vi "Main.vi"() -> ()   [LabVIEW 2018]
panel:
  in  "Air Dry Position Switch":bool
  in  "Main Wash Position Switch":bool
  in  "Under Body Wash Position Switch":bool
  in  "Economy Wash":bool
  in  "Deluxe Wash":bool
  out "Vehicle Out of Position":bool
  out "Air Dry":bool
  out "Clear Water Rinse":bool
  out "Main High Pressure Wash":bool
  out "Soap Aplication":bool
  out "Under Body Wash":bool
  in  "Stop":bool
  # "Purchase Selection"
  # "Car Wash Indicators"
  # "Car Wash Simulation Switches"
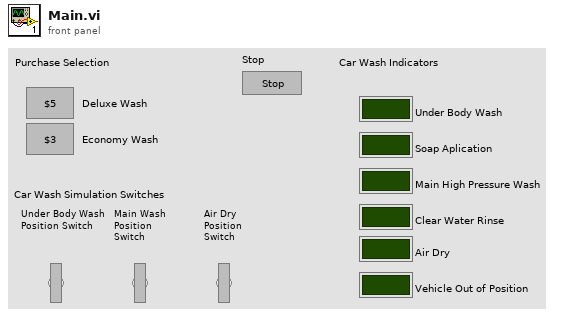
[diagram p1: front panel]
types:
  T1 = enum8{"Enabled", "Disabled", "Disabled and Grayed Out"}
  T2 = typedef "lista stnów.ctl" = enum16{"start", "ubderbody", "soap", "main", "main high", "clear water", "air", "air dry", "koniec"}
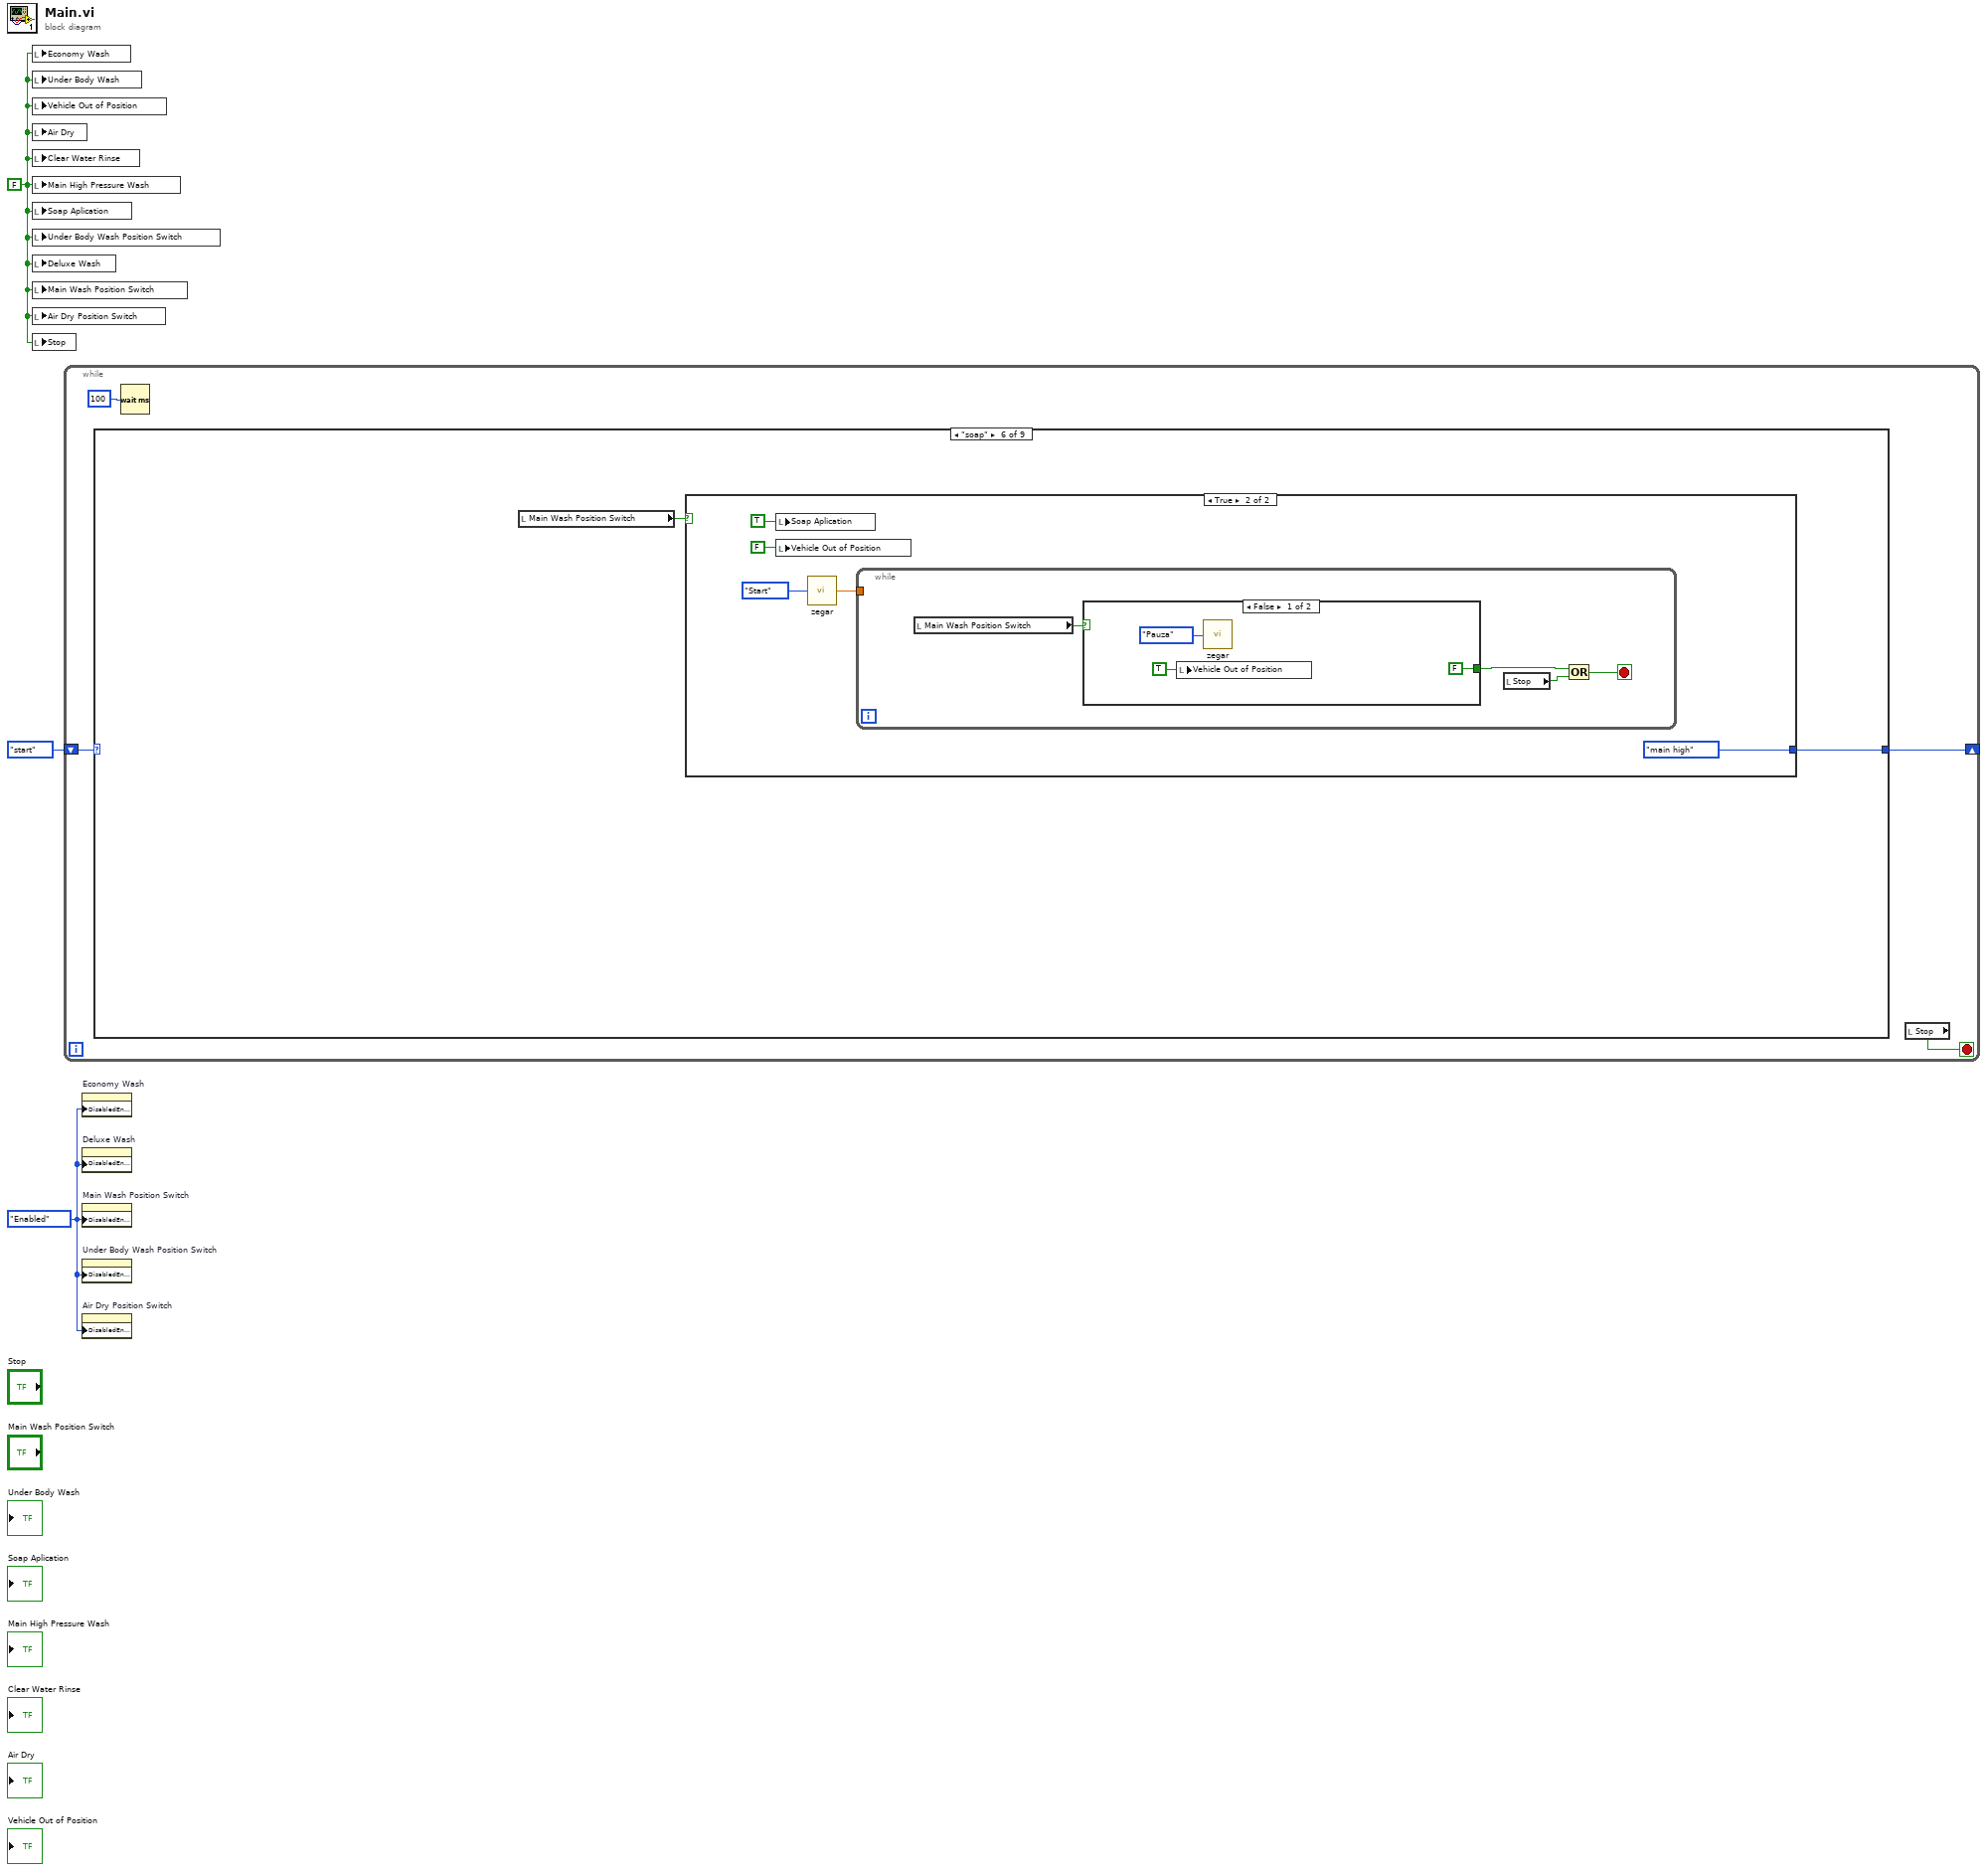
[diagram p0: block diagram]
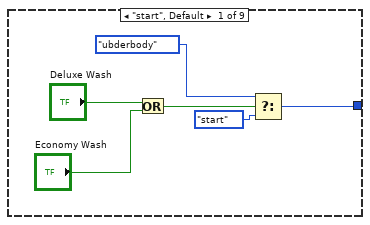
[diagram p2: hidden frame]
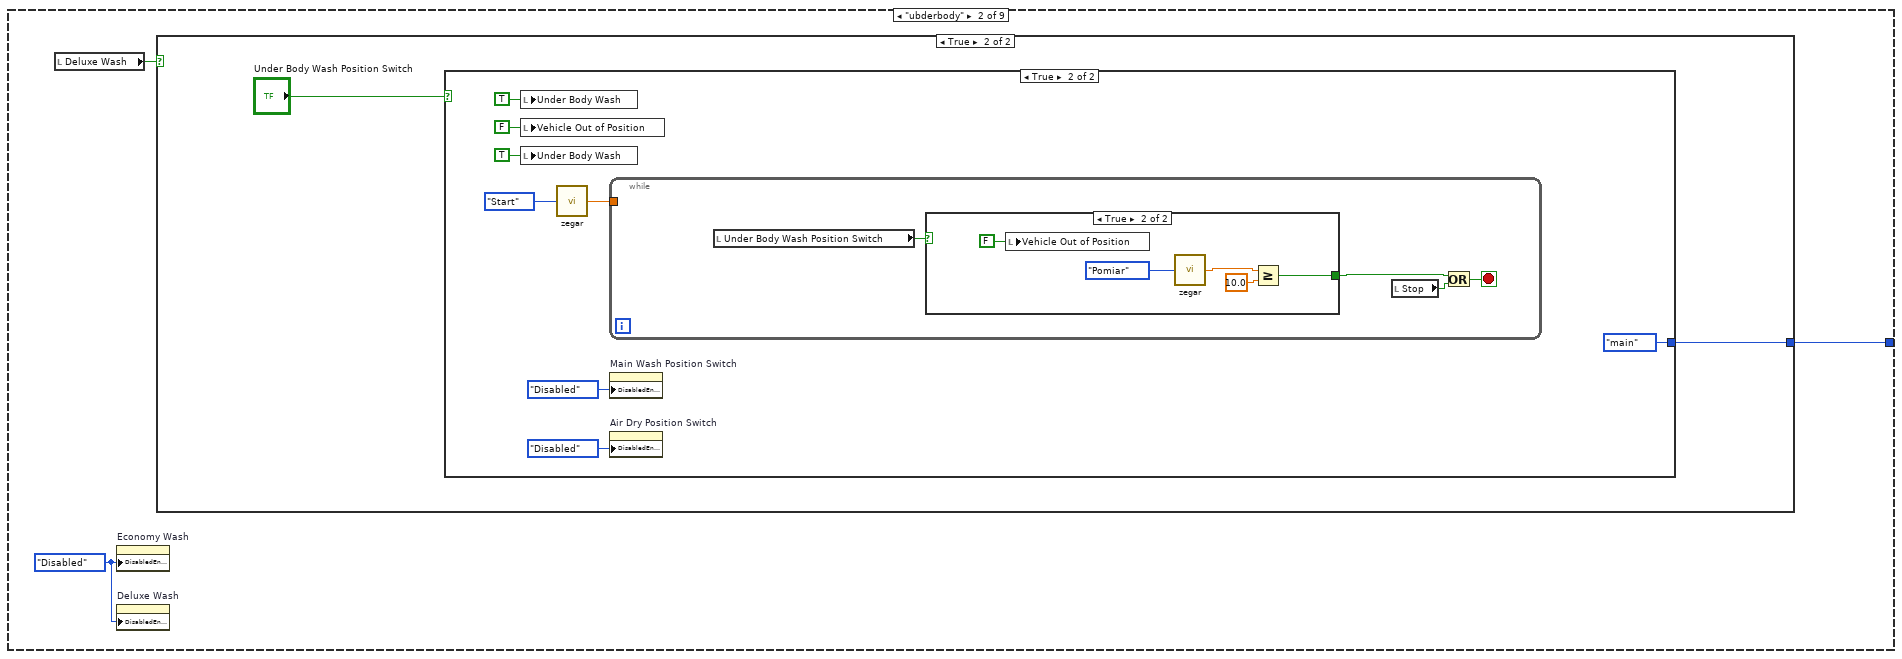
[diagram p3: hidden frame]
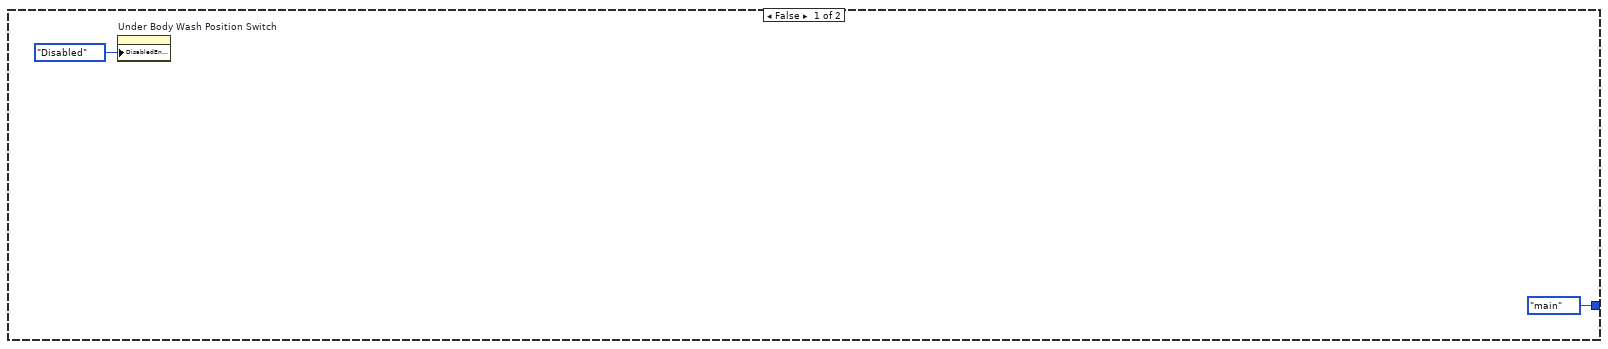
[diagram p4: hidden frame]
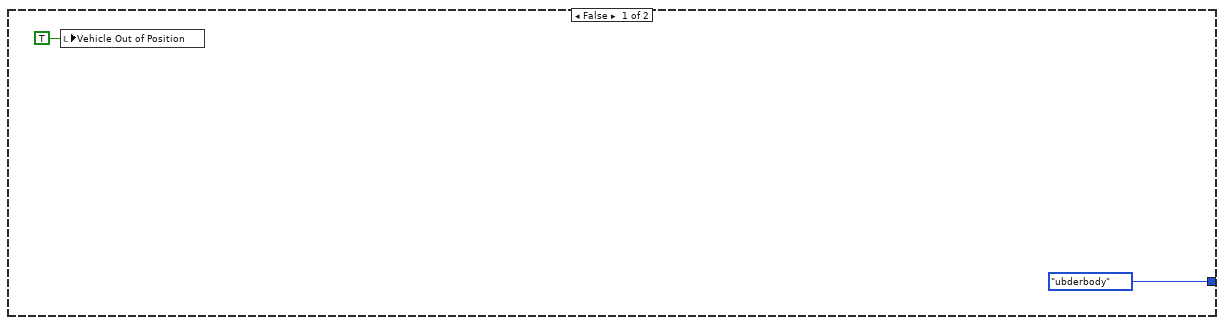
[diagram p5: hidden frame]
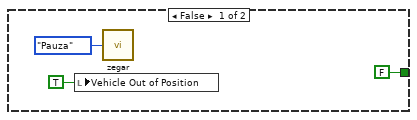
[diagram p6: hidden frame]
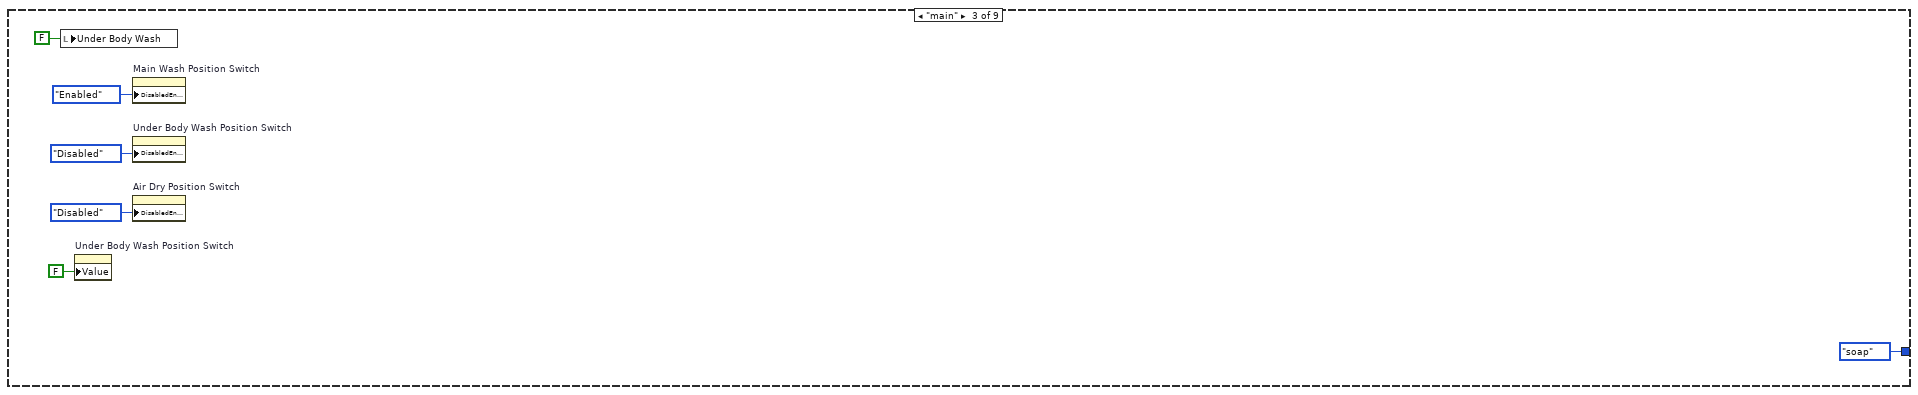
[diagram p7: hidden frame]
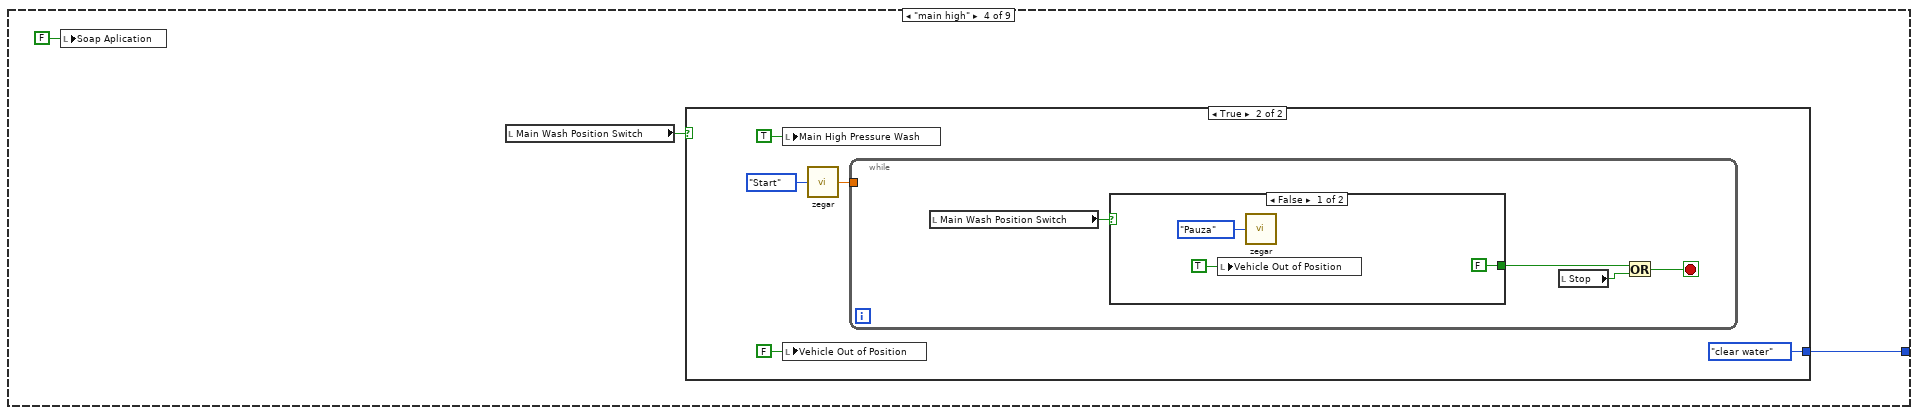
[diagram p8: hidden frame]
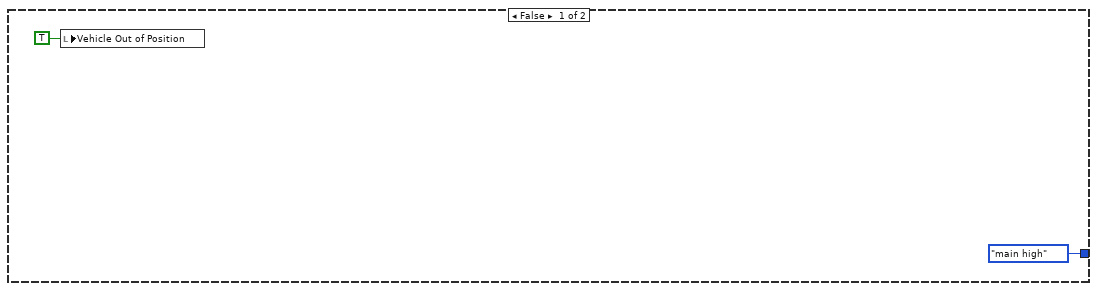
[diagram p9: hidden frame]
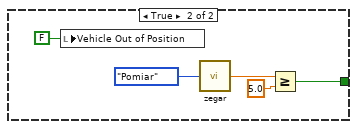
[diagram p10: hidden frame]
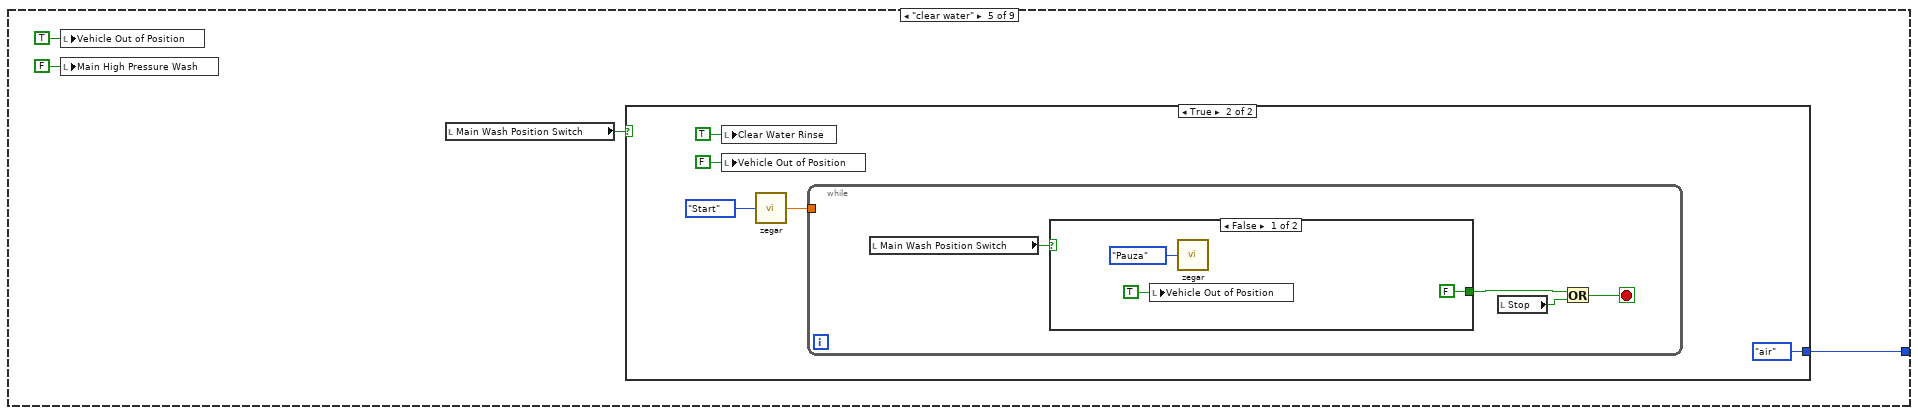
[diagram p11: hidden frame]
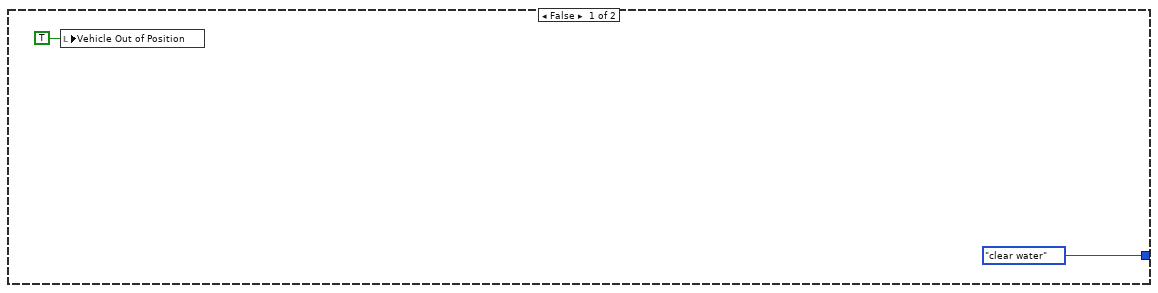
[diagram p12: hidden frame]
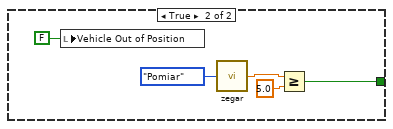
[diagram p13: hidden frame]
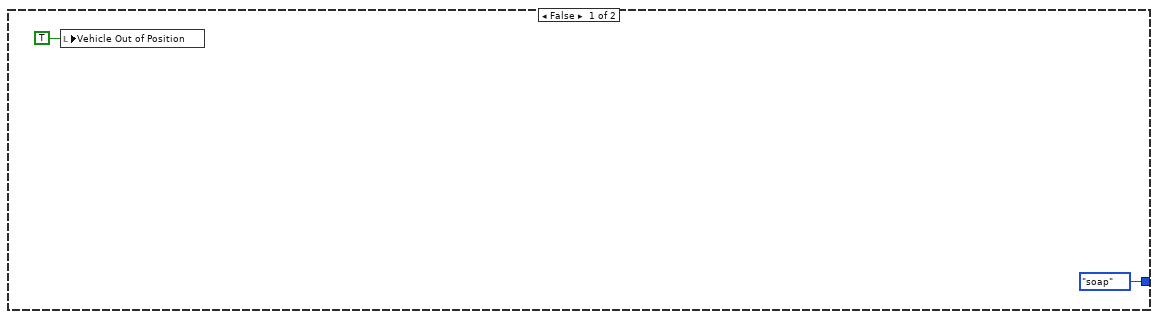
[diagram p14: hidden frame]
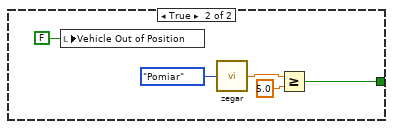
[diagram p15: hidden frame]
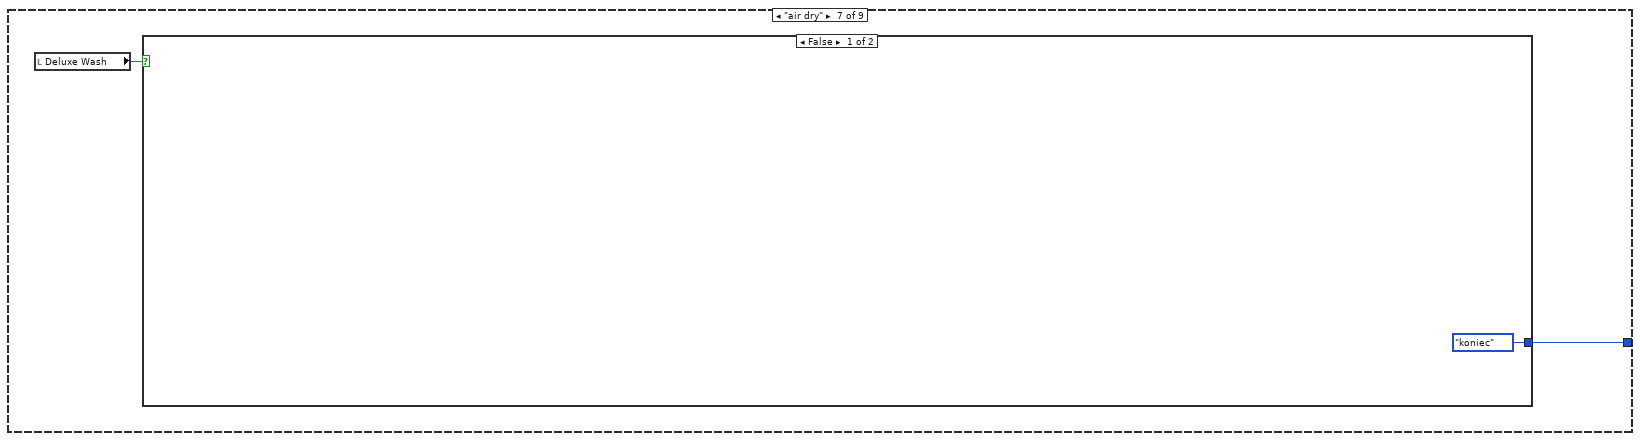
[diagram p16: hidden frame]
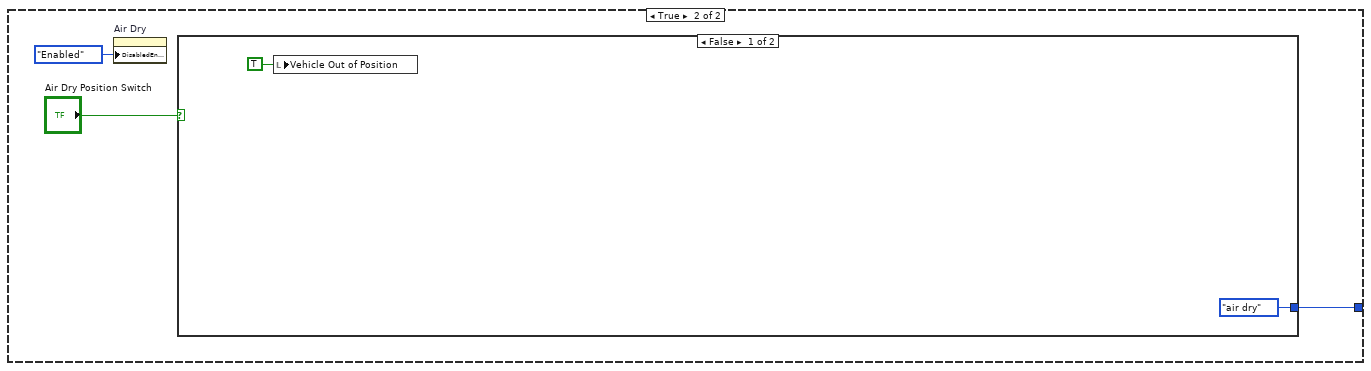
[diagram p17: hidden frame]
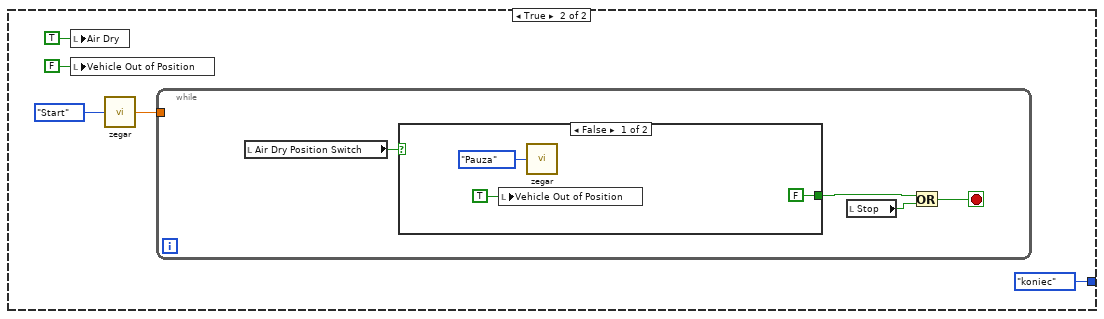
[diagram p18: hidden frame]
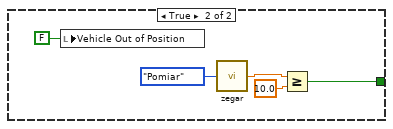
[diagram p19: hidden frame]
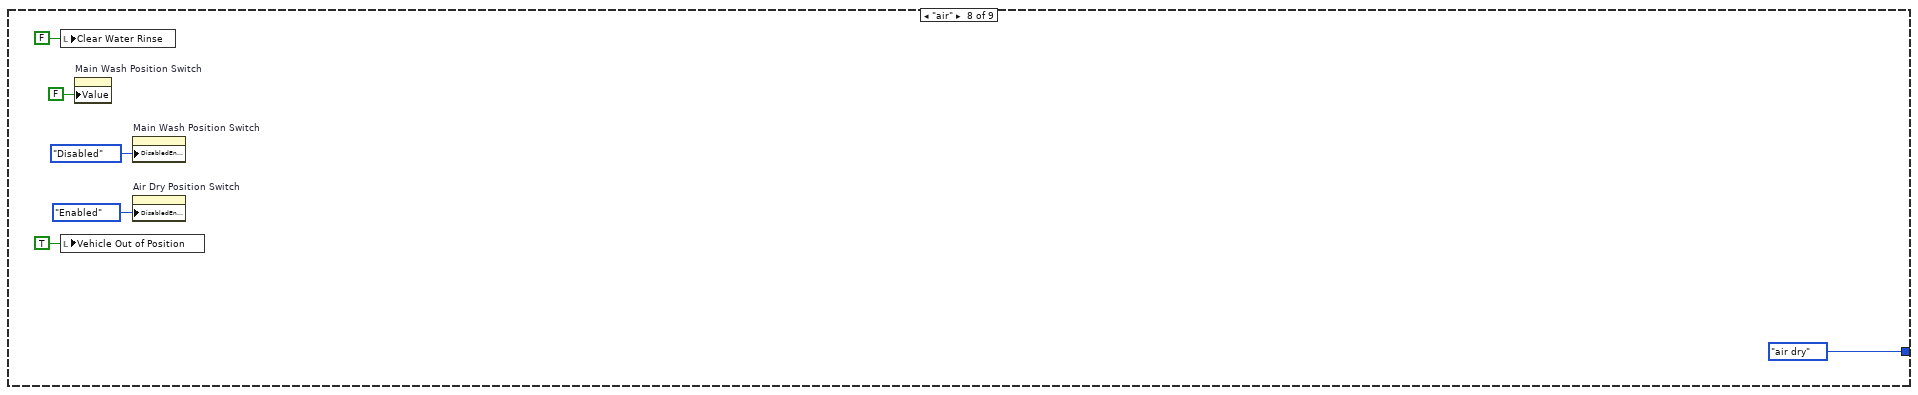
[diagram p20: hidden frame]
diagram:
  w1 = T1."Enabled" ("Disabled")
  w2 = FALSE
  n1 = local write "Economy Wash"(w2) -> ()
  n2 = local write "Under Body Wash"(w2) -> ()
  n3 = local write "Vehicle Out of Position"(w2) -> ()
  n4 = local write "Air Dry"(w2) -> ()
  n5 = local write "Clear Water Rinse"(w2) -> ()
  n6 = local write "Main High Pressure Wash"(w2) -> ()
  n7 = local write "Soap Aplication"(w2) -> ()
  n8 = local write "Under Body Wash Position Switch"(w2) -> ()
  n9 = local write "Deluxe Wash"(w2) -> ()
  n10 = local write "Main Wash Position Switch"(w2) -> ()
  n11 = local write "Air Dry Position Switch"(w2) -> ()
  n12 = local write "Stop"(w2) -> ()
  n13 = while {
    shift-right: [w5] -> _
    shift-left: lista_stnów."start" -> [w4]
    stop <- w7 stop-if-true
    n14 = case shown="\"soap\"" w4 {
      tunnel: [w8 w15 lista_stnów."soap" w49 w72 w94 w115 lista_stnów."air dry" lista_stnów."start"] -> w5
      frame "start", Default {
        n15 = Or(x="Deluxe Wash", y="Economy Wash") -> (x .or. y?=w11:bool)
        n16 = Select(t=lista_stnów."ubderbody", s=w11, f=lista_stnów."start") -> (s? t:f=w8:T2)
      }
      frame "ubderbody" {
        w14 = T1."Disabled" ("Disabled")
        n17 = local read "Deluxe Wash"() -> (w16:bool)
        n18 = property on="Economy Wash" class="Bool (strict)"("DisabledEnum"=w14) -> ()  [unwired: 2 in, 2 out]
        n19 = property on="Deluxe Wash" class="Bool (strict)"("DisabledEnum"=w14) -> ()  [unwired: 2 in, 2 out]
        n20 = case shown="True" w16 {
          tunnel: [lista_stnów."main" w19] -> w15
          frame False {
            n21 = property on="Under Body Wash Position Switch" class="Bool (strict)"("DisabledEnum"=T1."Disabled" ("Disabled")) -> ()  [unwired: 2 in, 2 out]
          }
          frame True {
            n22 = case shown="True" "Under Body Wash Position Switch" {
              tunnel: [lista_stnów."ubderbody" lista_stnów."main"] -> w19
              frame False {
                n23 = local write "Vehicle Out of Position"(TRUE ("Vehicle Out of Position 2")) -> ()
              }
              frame True {
                n24 = local write "Under Body Wash"(TRUE ("Under Body Wash")) -> ()
                n25 = local write "Vehicle Out of Position"(FALSE ("Vehicle Out of Position")) -> ()
                n26 = local write "Under Body Wash"(TRUE ("Under Body Wash")) -> ()
                n27 = call "zegar.vi"("zadanie"=enum16{"Start", "Pauza", "Pomiar"}."Start") -> ("x-y"=w26:dbl)
                n28 = while {
                  tunnel: w26 -> [_]
                  stop <- w31 stop-if-true
                  n29 = local read "Under Body Wash Position Switch"() -> (w34:bool)
                  n30 = case shown="True" w34 {
                    tunnel: [FALSE w39] -> w33
                    frame False {
                      n31 = local write "Vehicle Out of Position"(TRUE ("Vehicle Out of Position 2")) -> ()
                      n32 = call "zegar.vi"("zadanie"=enum16{"Start", "Pauza", "Pomiar"}."Pauza") -> ()  [unwired: 1 out]
                    }
                    frame True {
                      n33 = local write "Vehicle Out of Position"(FALSE ("Vehicle Out of Position")) -> ()
                      n34 = call "zegar.vi"("zadanie"=enum16{"Start", "Pauza", "Pomiar"}."Pomiar") -> ("x-y"=w41:dbl)
                      n35 = Greater Or Equal?(x=w41, y=10.0) -> (x >= y?=w39:bool)
                    }
                  }
                  n36 = local read "Stop"() -> (w32:bool)
                  n37 = Or(x=w33, y=w32) -> (x .or. y?=w31:bool)
                }
                n38 = property on="Main Wash Position Switch" class="Bool (strict)"("DisabledEnum"=T1."Disabled" ("Disabled")) -> ()  [unwired: 2 in, 2 out]
                n39 = property on="Air Dry Position Switch" class="Bool (strict)"("DisabledEnum"=T1."Disabled" ("Disabled")) -> ()  [unwired: 2 in, 2 out]
              }
            }
          }
        }
      }
      frame "main" {
        n40 = local write "Under Body Wash"(FALSE ("Under Body Wash")) -> ()
        n41 = property on="Under Body Wash Position Switch" class="Bool (strict)"("Value"=FALSE ("Main Wash Position Switch")) -> ()  [unwired: 2 in, 2 out]
        n42 = property on="Main Wash Position Switch" class="Bool (strict)"("DisabledEnum"=T1."Enabled" ("Disabled")) -> ()  [unwired: 2 in, 2 out]
        n43 = property on="Under Body Wash Position Switch" class="Bool (strict)"("DisabledEnum"=T1."Disabled" ("Disabled")) -> ()  [unwired: 2 in, 2 out]
        n44 = property on="Air Dry Position Switch" class="Bool (strict)"("DisabledEnum"=T1."Disabled" ("Disabled")) -> ()  [unwired: 2 in, 2 out]
      }
      frame "main high" {
        n45 = local write "Soap Aplication"(FALSE ("Under Body Wash")) -> ()
        n46 = local read "Main Wash Position Switch"() -> (w51:bool)
        n47 = case shown="True" w51 {
          tunnel: [lista_stnów."main high" lista_stnów."clear water"] -> w49
          frame False {
            n48 = local write "Vehicle Out of Position"(TRUE ("Vehicle Out of Position 2")) -> ()
          }
          frame True {
            n49 = local write "Main High Pressure Wash"(TRUE ("Under Body Wash")) -> ()
            n50 = local write "Vehicle Out of Position"(FALSE ("Vehicle Out of Position")) -> ()
            n51 = call "zegar.vi"("zadanie"=enum16{"Start", "Pauza", "Pomiar"}."Start") -> ("x-y"=w54:dbl)
            n52 = while {
              tunnel: w54 -> [_]
              stop <- w59 stop-if-true
              n53 = local read "Main Wash Position Switch"() -> (w62:bool)
              n54 = case shown="False" w62 {
                tunnel: [FALSE w67] -> w61
                frame False {
                  n55 = local write "Vehicle Out of Position"(TRUE ("Vehicle Out of Position")) -> ()
                  n56 = call "zegar.vi"("zadanie"=enum16{"Start", "Pauza", "Pomiar"}."Pauza") -> ()  [unwired: 1 out]
                }
                frame True {
                  n57 = local write "Vehicle Out of Position"(FALSE ("Vehicle Out of Position")) -> ()
                  n58 = call "zegar.vi"("zadanie"=enum16{"Start", "Pauza", "Pomiar"}."Pomiar") -> ("x-y"=w69:dbl)
                  n59 = Greater Or Equal?(x=w69, y=5.0) -> (x >= y?=w67:bool)
                }
              }
              n60 = local read "Stop"() -> (w60:bool)
              n61 = Or(x=w61, y=w60) -> (x .or. y?=w59:bool)
            }
          }
        }
      }
      frame "clear water" {
        n62 = local write "Vehicle Out of Position"(TRUE ("Vehicle Out of Position")) -> ()
        n63 = local write "Main High Pressure Wash"(FALSE ("Under Body Wash")) -> ()
        n64 = local read "Main Wash Position Switch"() -> (w74:bool)
        n65 = case shown="True" w74 {
          tunnel: [lista_stnów."clear water" lista_stnów."air"] -> w72
          frame False {
            n66 = local write "Vehicle Out of Position"(TRUE ("Vehicle Out of Position 2")) -> ()
          }
          frame True {
            n67 = local write "Clear Water Rinse"(TRUE ("Under Body Wash")) -> ()
            n68 = local write "Vehicle Out of Position"(FALSE ("Vehicle Out of Position")) -> ()
            n69 = call "zegar.vi"("zadanie"=enum16{"Start", "Pauza", "Pomiar"}."Start") -> ("x-y"=w77:dbl)
            n70 = while {
              tunnel: w77 -> [_]
              stop <- w82 stop-if-true
              n71 = local read "Main Wash Position Switch"() -> (w85:bool)
              n72 = case shown="False" w85 {
                tunnel: [FALSE w90] -> w84
                frame False {
                  n73 = local write "Vehicle Out of Position"(TRUE ("Vehicle Out of Position")) -> ()
                  n74 = call "zegar.vi"("zadanie"=enum16{"Start", "Pauza", "Pomiar"}."Pauza") -> ()  [unwired: 1 out]
                }
                frame True {
                  n75 = local write "Vehicle Out of Position"(FALSE ("Vehicle Out of Position")) -> ()
                  n76 = call "zegar.vi"("zadanie"=enum16{"Start", "Pauza", "Pomiar"}."Pomiar") -> ("x-y"=w92:dbl)
                  n77 = Greater Or Equal?(x=w92, y=5.0) -> (x >= y?=w90:bool)
                }
              }
              n78 = local read "Stop"() -> (w83:bool)
              n79 = Or(x=w84, y=w83) -> (x .or. y?=w82:bool)
            }
          }
        }
      }
      frame "soap" {
        n80 = local read "Main Wash Position Switch"() -> (w95:bool)
        n81 = case shown="True" w95 {
          tunnel: [lista_stnów."soap" lista_stnów."main high"] -> w94
          frame False {
            n82 = local write "Vehicle Out of Position"(TRUE ("Vehicle Out of Position 2")) -> ()
          }
          frame True {
            n83 = local write "Soap Aplication"(TRUE ("Under Body Wash")) -> ()
            n84 = local write "Vehicle Out of Position"(FALSE ("Vehicle Out of Position")) -> ()
            n85 = call "zegar.vi"("zadanie"=enum16{"Start", "Pauza", "Pomiar"}."Start") -> ("x-y"=w98:dbl)
            n86 = while {
              tunnel: w98 -> [_]
              stop <- w103 stop-if-true
              n87 = local read "Main Wash Position Switch"() -> (w106:bool)
              n88 = case shown="False" w106 {
                tunnel: [FALSE w111] -> w105
                frame False {
                  n89 = local write "Vehicle Out of Position"(TRUE ("Vehicle Out of Position")) -> ()
                  n90 = call "zegar.vi"("zadanie"=enum16{"Start", "Pauza", "Pomiar"}."Pauza") -> ()  [unwired: 1 out]
                }
                frame True {
                  n91 = local write "Vehicle Out of Position"(FALSE ("Vehicle Out of Position")) -> ()
                  n92 = call "zegar.vi"("zadanie"=enum16{"Start", "Pauza", "Pomiar"}."Pomiar") -> ("x-y"=w113:dbl)
                  n93 = Greater Or Equal?(x=w113, y=5.0) -> (x >= y?=w111:bool)
                }
              }
              n94 = local read "Stop"() -> (w104:bool)
              n95 = Or(x=w105, y=w104) -> (x .or. y?=w103:bool)
            }
          }
        }
      }
      frame "air dry" {
        n96 = local read "Deluxe Wash"() -> (w116:bool)
        n97 = case shown="False" w116 {
          tunnel: [lista_stnów."koniec" w119] -> w115
          frame False {
          }
          frame True {
            n98 = property on="Air Dry" class="Bool (strict)"("DisabledEnum"=T1."Enabled" ("Disabled")) -> ()  [unwired: 2 in, 2 out]
            n99 = case shown="False" "Air Dry Position Switch" {
              tunnel: [lista_stnów."air dry" lista_stnów."koniec"] -> w119
              frame False {
                n100 = local write "Vehicle Out of Position"(TRUE ("Vehicle Out of Position 2")) -> ()
              }
              frame True {
                n101 = local write "Air Dry"(TRUE ("Under Body Wash")) -> ()
                n102 = local write "Vehicle Out of Position"(FALSE ("Vehicle Out of Position")) -> ()
                n103 = call "zegar.vi"("zadanie"=enum16{"Start", "Pauza", "Pomiar"}."Start") -> ("x-y"=w123:dbl)
                n104 = while {
                  tunnel: w123 -> [_]
                  stop <- w128 stop-if-true
                  n105 = local read "Air Dry Position Switch"() -> (w131:bool)
                  n106 = case shown="False" w131 {
                    tunnel: [FALSE w136] -> w130
                    frame False {
                      n107 = local write "Vehicle Out of Position"(TRUE ("Vehicle Out of Position")) -> ()
                      n108 = call "zegar.vi"("zadanie"=enum16{"Start", "Pauza", "Pomiar"}."Pauza") -> ()  [unwired: 1 out]
                    }
                    frame True {
                      n109 = local write "Vehicle Out of Position"(FALSE ("Vehicle Out of Position")) -> ()
                      n110 = call "zegar.vi"("zadanie"=enum16{"Start", "Pauza", "Pomiar"}."Pomiar") -> ("x-y"=w138:dbl)
                      n111 = Greater Or Equal?(x=w138, y=10.0) -> (x >= y?=w136:bool)
                    }
                  }
                  n112 = local read "Stop"() -> (w129:bool)
                  n113 = Or(x=w130, y=w129) -> (x .or. y?=w128:bool)
                }
              }
            }
          }
        }
      }
      frame "air" {
        n114 = local write "Clear Water Rinse"(FALSE ("Under Body Wash")) -> ()
        n115 = local write "Vehicle Out of Position"(TRUE ("Vehicle Out of Position")) -> ()
        n116 = property on="Main Wash Position Switch" class="Bool (strict)"("Value"=FALSE ("Main Wash Position Switch")) -> ()  [unwired: 2 in, 2 out]
        n117 = property on="Main Wash Position Switch" class="Bool (strict)"("DisabledEnum"=T1."Disabled" ("Disabled")) -> ()  [unwired: 2 in, 2 out]
        n118 = property on="Air Dry Position Switch" class="Bool (strict)"("DisabledEnum"=T1."Enabled" ("Disabled")) -> ()  [unwired: 2 in, 2 out]
      }
      frame "koniec" {
        w147 = T1."Enabled" ("Disabled")
        w148 = FALSE
        n119 = local write "Stop"(w148) -> ()
        n120 = local write "Air Dry"(w148) -> ()
        n121 = local write "Clear Water Rinse"(w148) -> ()
        n122 = local write "Main High Pressure Wash"(w148) -> ()
        n123 = local write "Economy Wash"(w148) -> ()
        n124 = local write "Soap Aplication"(w148) -> ()
        n125 = local write "Under Body Wash Position Switch"(w148) -> ()
        n126 = local write "Deluxe Wash"(w148) -> ()
        n127 = local write "Main Wash Position Switch"(w148) -> ()
        n128 = local write "Under Body Wash"(w148) -> ()
        n129 = local write "Vehicle Out of Position"(w148) -> ()
        n130 = local write "Air Dry Position Switch"(w148) -> ()
        n131 = property on="Economy Wash" class="Bool (strict)"("DisabledEnum"=w147) -> ()  [unwired: 2 in, 2 out]
        n132 = property on="Deluxe Wash" class="Bool (strict)"("DisabledEnum"=w147) -> ()  [unwired: 2 in, 2 out]
        n133 = property on="Main Wash Position Switch" class="Bool (strict)"("DisabledEnum"=w147) -> ()  [unwired: 2 in, 2 out]
        n134 = property on="Under Body Wash Position Switch" class="Bool (strict)"("DisabledEnum"=w147) -> ()  [unwired: 2 in, 2 out]
        n135 = property on="Air Dry Position Switch" class="Bool (strict)"("DisabledEnum"=w147) -> ()  [unwired: 2 in, 2 out]
      }
    }
    n136 = Wait (ms)(milliseconds to wait=u32 100) -> ()  [unwired: 1 out]
    n137 = local read "Stop"() -> (w7:bool)
  }
  n138 = property on="Economy Wash" class="Bool (strict)"("DisabledEnum"=w1) -> ()  [unwired: 2 in, 2 out]
  n139 = property on="Deluxe Wash" class="Bool (strict)"("DisabledEnum"=w1) -> ()  [unwired: 2 in, 2 out]
  n140 = property on="Main Wash Position Switch" class="Bool (strict)"("DisabledEnum"=w1) -> ()  [unwired: 2 in, 2 out]
  n141 = property on="Under Body Wash Position Switch" class="Bool (strict)"("DisabledEnum"=w1) -> ()  [unwired: 2 in, 2 out]
  n142 = property on="Air Dry Position Switch" class="Bool (strict)"("DisabledEnum"=w1) -> ()  [unwired: 2 in, 2 out]
